vi "manual_action-block.vi"(6 "timeout_s":dbl=-1.0 format="%#_13g", 8 "error in (no error)":errorcluster, 10 "data":variant, 11 "step":string) -> (0 "error out":errorcluster)   [LabVIEW 2015, in "lv-recipe-machine.lvlib"]
uses:
  lv-recipe-machine.lvlib
  _controls/error.ctl
  _controls/manual_state.ctl
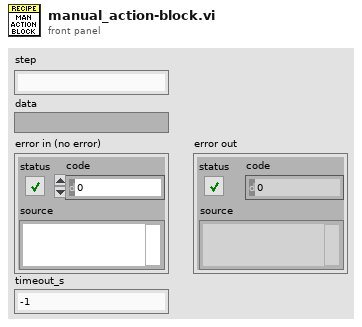
[diagram p1: front panel]
types:
  T1 = typedef "lv-recipe-machine.lvlib/error.ctl" = enum16{"<error>", "bad_command", "command_queue_timeout", "stop_notifier_timeout", "die_command_timeout", "not_in_manual_mode", "not_in_automatic_mode", "not_in_automatic_idle", "not_in_automatic_running", "not_in_automatic_paused", "automatic_step_not_found", "manual_action_not_found", "automatic_not_transition_vi", "transition_step_not_found", "unsupported_vi_type", "manual_block_timeout", "<null>"}
  T2 = typedef "lv-recipe-machine.lvlib/manual_state.ctl" = enum16{"<manual_state>", "failed", "action", "running", "idle", "<null>"}
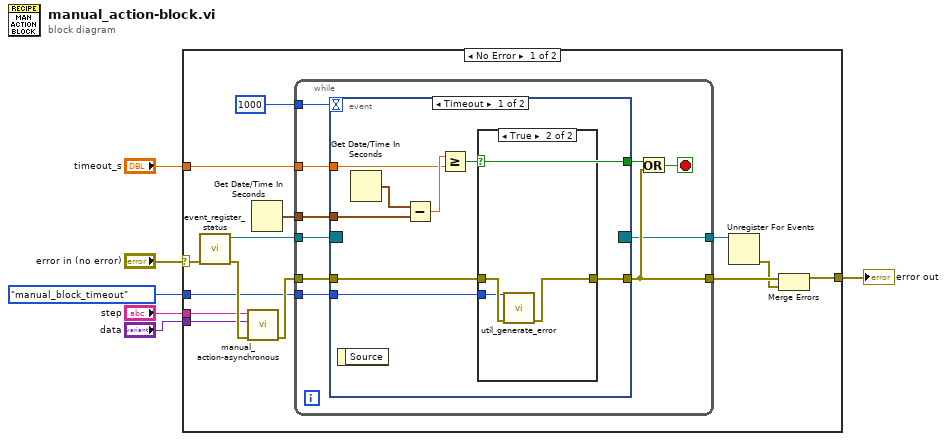
[diagram p0: block diagram]
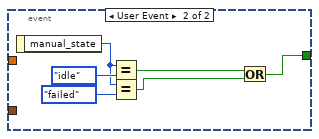
[diagram p3: hidden frame]
diagram:
  n1 = case shown="No Error" "error in (no error)" {
    selector: "error in (no error)" -> [w18 w49]
    tunnel: "data" -> [w17 _]
    tunnel: "step" -> [w16 _]
    tunnel: "timeout_s" -> [w13 _]
    tunnel: [w9 w49] -> w2
    tunnel: error."manual_block_timeout" ("error") -> [w7 _]
    frame No Error {
      n2 = call "event_register_status.vi"("error in (no error)"=w18) -> ("error out"=w20:errorcluster, "status_event_registration"=w14:refnum<event-registration>)  [unwired: 9 in]
      n3 = call "manual_action-asynchronous.vi"("error in (no error)"=w20, "data"=w17, "step"=w16) -> ("error out"=w19:errorcluster)  [unwired: 8 in]
      n4 = Get Date/Time In Seconds() -> (seconds since 1Jan1904=w11:timestamp)
      n5 = while {
        tunnel: w19 -> [w30]
        tunnel: [w29] -> w12
        tunnel: 1000 -> [w27]
        tunnel: w14 -> [w26]
        tunnel: w13 -> [w25]
        tunnel: w11 -> [w24]
        tunnel: [w22] -> w10
        tunnel: w7 -> [w21]
        stop <- w28 stop-if-true
        n6 = event shown="[0] Timeout" {
          selector: w26 -> [_ _]
          dyn-events: [_ _] -> w22
          timeout: w27 -> [_ _]
          tunnel: w30 -> [w32 _]
          tunnel: [w31 _] -> w29
          tunnel: w25 -> [w35 _]
          tunnel: w24 -> [w37 _]
          tunnel: [w34 w43] -> w23
          tunnel: w21 -> [w33 _]
          event Timeout {
            n7 = event-data() -> ()  [unwired: 1 in, 1 out]
            n8 = Get Date/Time In Seconds() -> (seconds since 1Jan1904=w38:timestamp)
            n9 = Subtract(x=w38, y=w37) -> (x-y=w36:dbl)
            n10 = Greater Or Equal?(x=w36, y=w35) -> (x >= y?=w34:bool)
            n11 = case shown="True" w34 {
              tunnel: w33 -> [_ w40]
              tunnel: w32 -> [w39 w42]
              tunnel: [w39 w41] -> w31
              frame False {
              }
              frame True {
                n12 = call "util_generate_error.vi"("error in (no error)"=w42, "error"=w40) -> ("error out"=w41:errorcluster)  [unwired: 9 in]
              }
            }
          }
          event User Event {
            n13 = event-data() -> ("manual_state"=w47:T2)  [unwired: 1 in]
            n14 = Equal?(x=w47, y=manual_state."idle") -> (x = y?=w45:bool)
            n15 = Equal?(x=w47, y=manual_state."failed") -> (x = y?=w44:bool)
            n16 = Or(x=w45, y=w44) -> (x .or. y?=w43:bool)
          }
        }
        n17 = Or(x=w23, y=w29) -> (x .or. y?=w28:bool)
      }
      n18 = Unregister For Events(event registration refnum=w10) -> (error out=w8:errorcluster)  [unwired: 1 in]
      n19 = Merge Errors(w12, w8) -> (w9:errorcluster)
    }
    frame Error {
    }
  }
  "error out" <- w2
